vi "Ex1 head.vi"() -> ()   [LabVIEW 2013]
panel:
  in  "Nod":bool=TRUE
  in  "Send":bool=TRUE
  in  "stop":bool
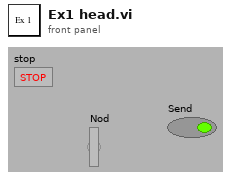
[diagram p1: front panel]
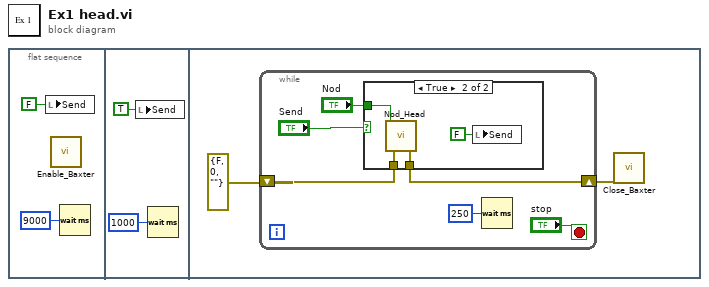
[diagram p0: block diagram]
diagram:
  n1 = flat-sequence {
    frame #0 {
      n2 = local write "Send"(FALSE ("Send")) -> ()
      n3 = call "Enable_Baxter.vi"() -> ()  [unwired: 4 in, 1 out]
      n4 = Wait (ms)(milliseconds to wait=u32 9000) -> ()  [unwired: 1 out]
    }
    frame #1 {
      n5 = local write "Send"(TRUE ("Nod")) -> ()
      n6 = Wait (ms)(milliseconds to wait=u32 1000) -> ()  [unwired: 1 out]
    }
    frame #2 {
      n7 = while {
        shift-right: [w9] -> w6
        shift-left: errorcluster {"status"=FALSE, "code"=0, "source"=""} ("error out") -> [w10]
        stop <- "stop" stop-if-true
        n8 = case shown="True" "Send" {
          tunnel: w10 -> [w13 w17]
          tunnel: [w13 w16] -> w9
          tunnel: "Nod" -> [_ w14]
          frame False {
          }
          frame True {
            n9 = call "Nod_Head.vi"("error in"=w17, "State"=w14) -> ("error out"=w16:errorcluster)  [unwired: 2 in]
            n10 = local write "Send"(FALSE ("Nod")) -> ()
          }
        }
        n11 = Wait (ms)(milliseconds to wait=u32 250) -> ()  [unwired: 1 out]
      }
      n12 = call "Close_Baxter.vi"("error in"=w6) -> ()  [unwired: 3 in, 1 out]
    }
  }
